vi "Main.vi"(8 "error in (no error)":errorcluster, 11 "ModuleAdmin":refnum<class "ModuleAdmin.lvclass">) -> ()   [LabVIEW 2018, in "SensorPlugins.lvlib"]
uses:
  SensorPlugins.lvlib
  <userlib>/NIST/ModuleAdminLib/ModuleAdmin/ModuleAdmin.lvclass
  C:/Program Files (x86)/National Instruments/LabVIEW 2018/user.lib/NIST/ModuleAdminLib/ModuleAdminBase/ModuleAdminBase.lvclass
  SensorBaseClass/SensorBase.lvclass
  C:/Program Files (x86)/National Instruments/LabVIEW 2018/user.lib/NIST/BaseClasses/BasePlugin_class/BasePlugin.lvclass
  SensorShared/clStopArgument.ctl
  <userlib>/NIST/ModuleAdminLib/ModuleAdmin/ModuleAdmin.lvclass/ModuleAdmin.ctl
  <userlib>/NIST/BaseClasses/BasePlugin_class/BasePlugin.lvclass/BasePlugin.ctl
  <vilib>/Utility/error.llb/DialogType.ctl
  <userlib>/NIST/ModuleAdminLib/ModuleAdmin/Accessors/Read ShowPanel_.vi
  <userlib>/NIST/ModuleAdminLib/ModuleAdmin/Accessors/Write ShowPanel_.vi
  <userlib>/NIST/BaseClasses/BasePlugin_class/Accessors/Write PluginIniFilePath.vi
  <userlib>/NIST/BaseClasses/BasePlugin_class/Accessors/Read PluginIniFilePath.vi
  <userlib>/NIST/ModuleAdminLib/ModuleAdmin/Accessors/Read CloneRegRef.vi
  <vilib>/Utility/error.llb/Error Cluster From Error Code.vi
  <vilib>/ErrorRing/Error Ring.xnode
  <userlib>/NIST/ModuleAdminLib/CloneRegistration/CloneRegistration.lvclass
  SensorShared/SensorShared.lvlib
  <userlib>/NIST/BaseClasses/Object_class/BaseObject.lvclass
  <userlib>/NIST/ModuleAdminLib/ModuleAdmin.lvlib
panel:
  out "error out":errorcluster
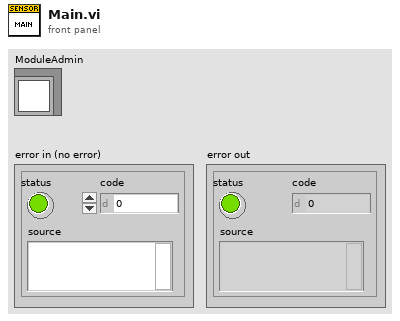
[diagram p1: front panel]
types:
  T1 = typedef "SensorShared.lvlib/clRequestEvents.ctl" = cluster{"StopRequest":refnum<user-event>, "PathToINI":refnum<user-event>, " LoadPlugin":refnum<user-event>, "ShowPanel":refnum<user-event>, "StartData":refnum<user-event>, "StopData":refnum<user-event>, "WriteConfig":refnum<user-event>, "ReadConfig":refnum<user-event>, "WriteEvtSignal":refnum<user-event>, "Configure":refnum<user-event>}
  T2 = typedef "SensorShared.lvlib/clBroadcastEvents.ctl" = cluster{"DidInit":refnum<user-event>, "StatusUpdate":refnum<user-event>, "ErrorReport":refnum<user-event>, "DidStop":refnum<user-event>, "PathToINI":refnum<user-event>, "SensorReport":refnum<user-event>, "SensorConfig":refnum<user-event>}
  T3 = typedef "SensorShared.lvlib/clStopArgument.ctl" = cluster{"Exit via Stop Module Req?":bool, "Wait for Module to stop?":bool, "ModuleAdmin":refnum<class "ModuleAdmin.lvclass">}
  T4 = enum32{"Invalid", "Standard", "Closed", "Hidden", "Minimized", "Maximized"}
  T5 = typedef "SensorShared.lvlib/clSensorData.ctl" = cluster{"SensorType":string, "SensorData":variant}
  T6 = typedef "DialogType.ctl" = u16
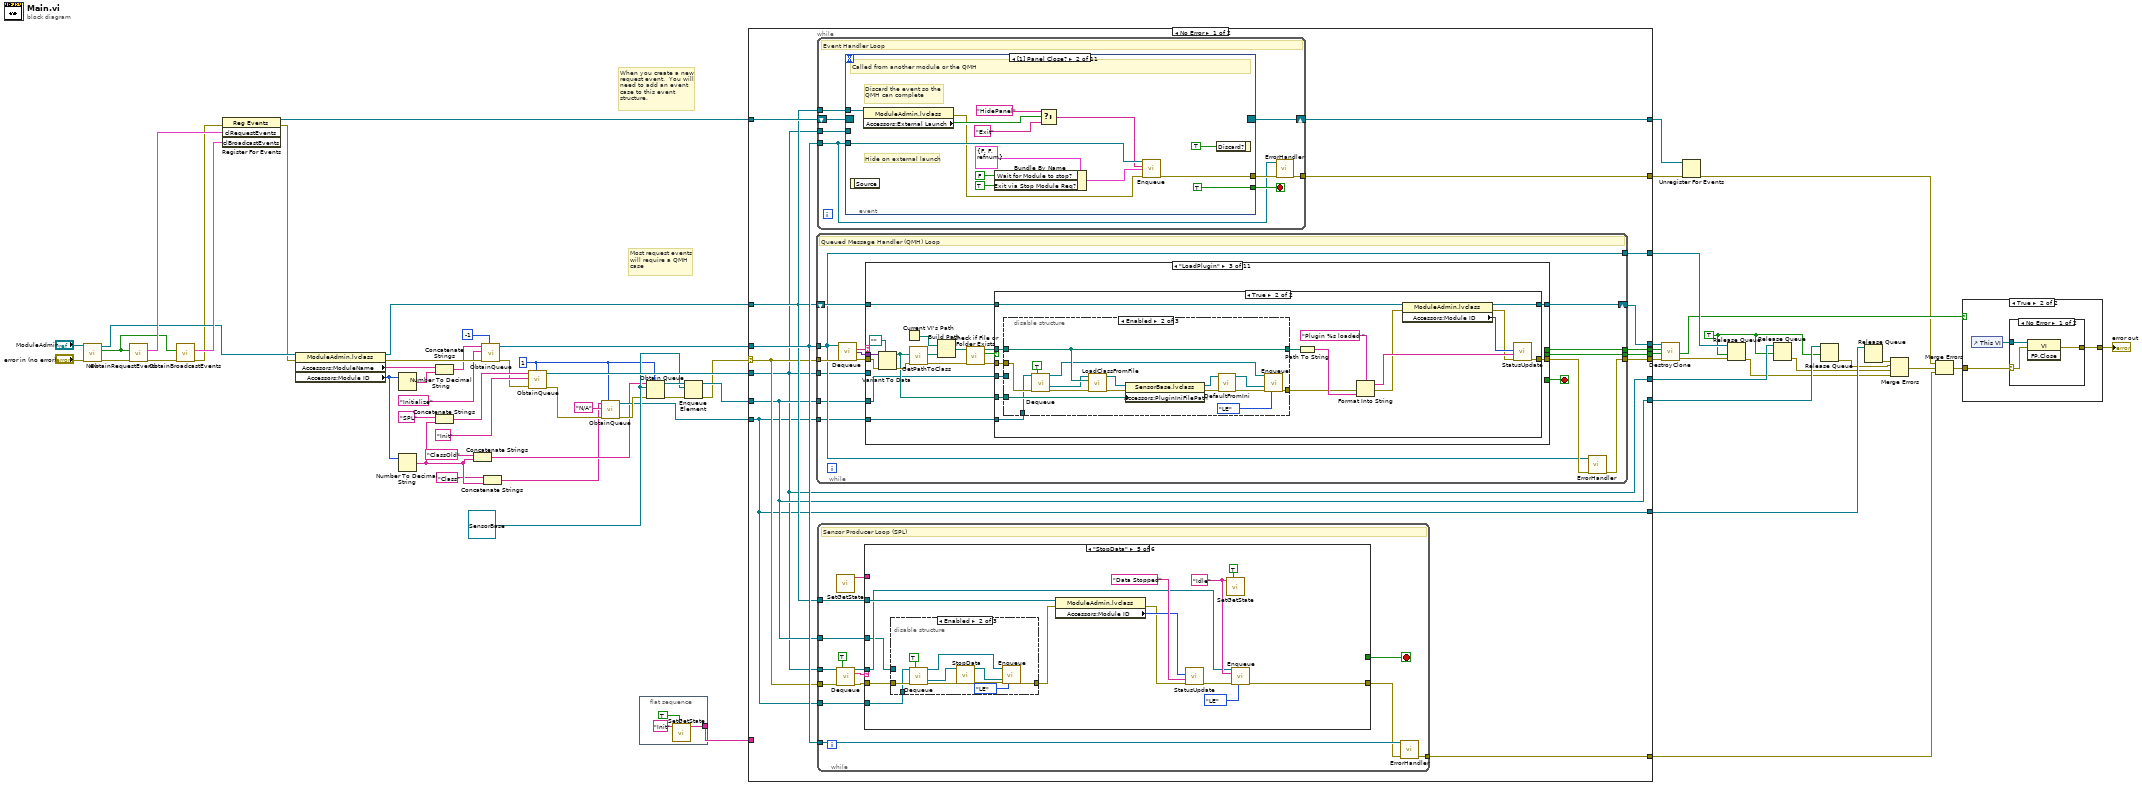
[diagram p0: block diagram]
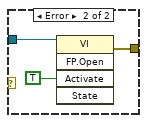
[diagram p3: hidden frame]
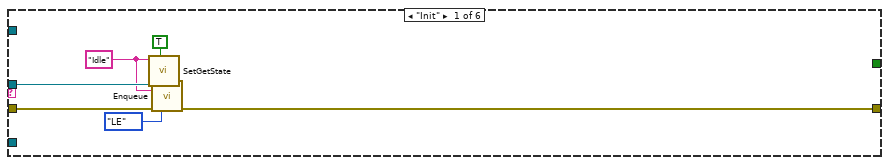
[diagram p4: hidden frame]
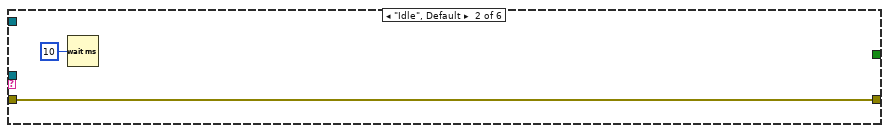
[diagram p5: hidden frame]
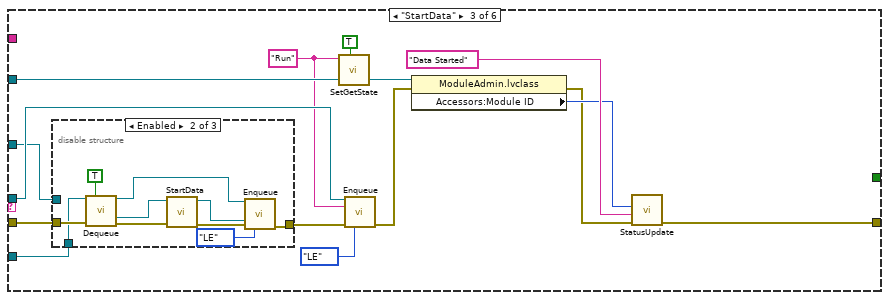
[diagram p6: hidden frame]
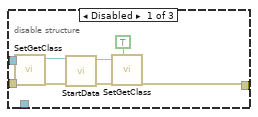
[diagram p7: hidden frame]
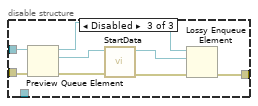
[diagram p8: hidden frame]
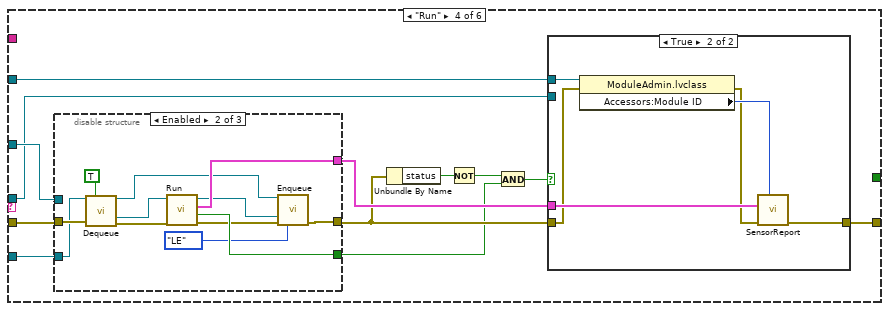
[diagram p9: hidden frame]
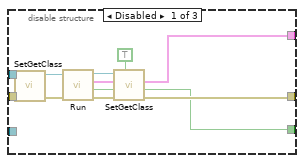
[diagram p10: hidden frame]
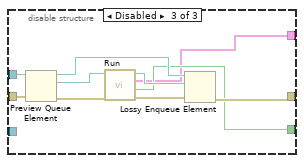
[diagram p11: hidden frame]
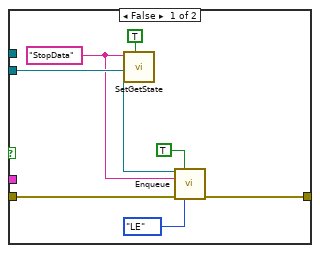
[diagram p12: hidden frame]
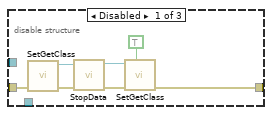
[diagram p13: hidden frame]
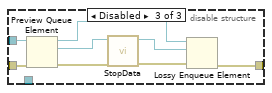
[diagram p14: hidden frame]
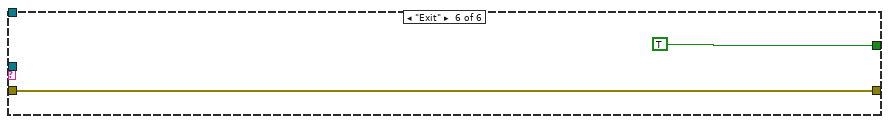
[diagram p15: hidden frame]
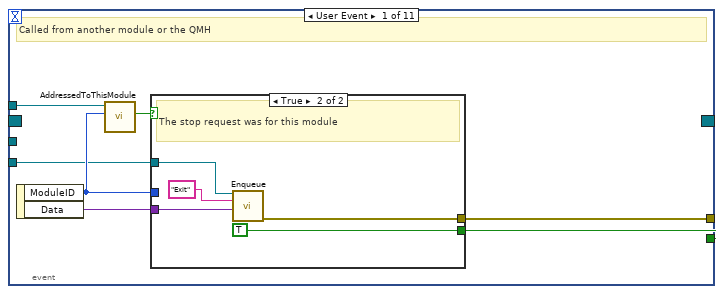
[diagram p16: hidden frame]
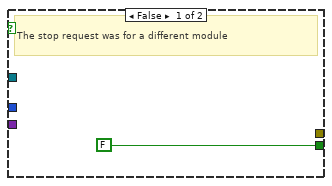
[diagram p17: hidden frame]
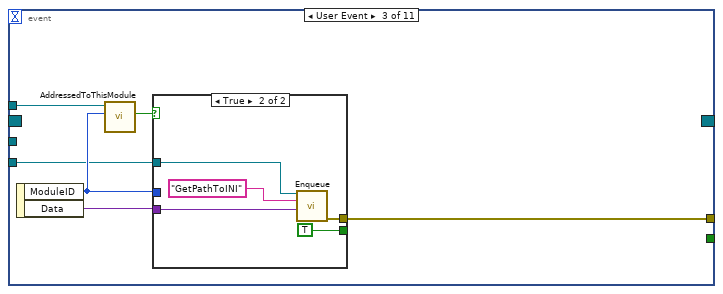
[diagram p18: hidden frame]
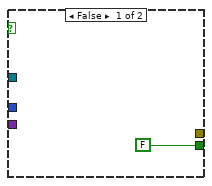
[diagram p19: hidden frame]
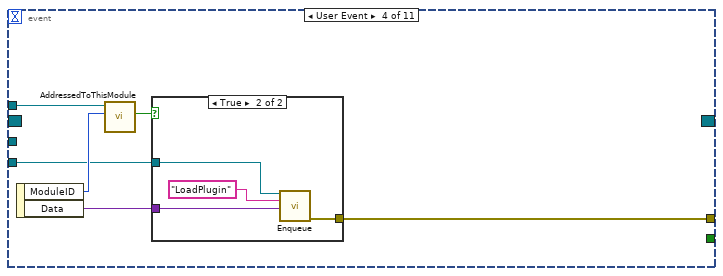
[diagram p20: hidden frame]
diagram:
  w16 = TRUE ("force destroy? (F)")
  w22 = refnum<class "SensorBase.lvclass"> refnum ("MyPlugins.lvlib:MyPluginsBase.lvclass")
  w14 = 1 ("Queue size (-1, unlimited)")
  # "Most request events\nwill require a QMH\ncase"
  # "When you create a new request event.  You will need to add an event case to this event structure."
  n1 = call <userlib>:"New.vi"("error in (no error)"="error in (no error)", "ModuleAdmin"="ModuleAdmin") -> ("error out"=w61:errorcluster, "First?"=w57:bool, "ModuleAdmin"=w42:refnum<class "ModuleAdmin.lvclass">)  [unwired: 6 in, 1 out]
  n2 = call "ObtainRequestEvents.vi"("error in (no error)"=w61, "CreateNew (F)"=w57) -> ("error out"=w56:errorcluster, "clRequestEvents"=w60:T1)  [unwired: 8 in]
  n3 = call "ObtainBroadcastEvents.vi"("error in (no error)"=w56, "CreateNew? (F)"=w57) -> ("error out"=w29:errorcluster, "clBroadcastEvents"=w55:T2)  [unwired: 8 in]
  n4 = register-events(error in=w29, w60, w55) -> (reference out=w54:refnum<event-registration>, error out=w28:errorcluster)  [unwired: 1 in]
  n5 = property class="ModuleAdmin.lvclass"(reference=w42, error in=w28) -> (reference out=w19:refnum<class "ModuleAdmin.lvclass">, error out=w44:errorcluster, "Accessors:ModuleName"=w40:string, "Accessors:Module ID"=w32:i32)
  n6 = Number To Decimal String(number=w32) -> (decimal integer string=w39:string)  [unwired: 1 in]
  n7 = Number To Decimal String(number=w32) -> (decimal integer string=w4:string)  [unwired: 1 in]
  n8 = Concatenate Strings(w40, w39) -> (w38:string)
  n9 = Concatenate Strings("SPL" ("Initial Message"), w4) -> (w34:string)
  n10 = Concatenate Strings("ClassOld" ("Initial Message"), w4) -> (w2:string)
  n11 = call "ObtainQueue.vi"("Queue size (-1, unlimited)"=-1, "error in (no error)"=w44, "Initial Message"="Initialize", "Queue Name"=w38) -> ("error out"=w33:errorcluster, "MessageQueue"=w59:refnum<queue>)  [unwired: 6 in]
  n12 = Concatenate Strings("Class" ("Initial Message"), w4) -> (w1:string)
  n13 = call "ObtainQueue.vi"("Queue size (-1, unlimited)"=w14, "error in (no error)"=w33, "Initial Message"="Init", "Queue Name"=w34) -> ("error out"=w15:errorcluster, "MessageQueue"=w30:refnum<queue>)  [unwired: 6 in]
  n14 = call "ObtainQueue.vi"("Queue size (-1, unlimited)"=w14, "error in (no error)"=w15, "Initial Message"="N/A", "Queue Name"=w1) -> ("error out"=w13:errorcluster, "MessageQueue"=w12:refnum<queue>)  [unwired: 6 in]
  n15 = flat-sequence {
    tunnel: [w64] -> w20
    frame #0 {
      n16 = call "SetGetState.vi"("Set (f)"=TRUE, "State In"="Init") -> ("State Out"=w64:string)  [unwired: 9 in]
    }
  }
  n17 = Obtain Queue(max queue size (-1, unlimited)=w14, name (unnamed)=w2, element data type=w22, error in (no error)=w13) -> (queue out=w24:refnum<queue>, error out=w26:errorcluster)  [unwired: 1 in, 1 out]
  n18 = Enqueue Element(queue=w24, element=w22, error in (no error)=w26) -> (queue out=w23:refnum<queue>, error out=w21:errorcluster)  [unwired: 1 in, 1 out]
  n19 = case shown="No Error" w21 {
    selector: w21 -> [w70 w737]
    tunnel: w59 -> [w74 w733]
    tunnel: w19 -> [w72 w734]
    tunnel: [w81 w735] -> w53
    tunnel: [w80 w733] -> w58
    tunnel: w54 -> [w79 w729]
    tunnel: [w78 w732] -> w51
    tunnel: [w77 _] -> w50
    tunnel: [w76 _] -> w49
    tunnel: [w75 _] -> w47
    tunnel: [w73 _] -> w27
    tunnel: [w71 w729] -> w46
    tunnel: w30 -> [w68 w726]
    tunnel: w23 -> [w69 w725]
    tunnel: w20 -> [_ _]
    tunnel: [w68 w726] -> w18
    tunnel: [w69 w725] -> w17
    tunnel: w12 -> [w67 w724]
    tunnel: [w67 w724] -> w10
    frame No Error {
      n20 = while {
        tunnel: w74 -> [w367]
        tunnel: w70 -> [w376]
        tunnel: [w369] -> w81
        tunnel: [w367] -> w80
        tunnel: [w371] -> w77
        tunnel: [w370] -> w76
        shift-right: [w366] -> w78
        shift-left: w72 -> [w372]
        tunnel: w69 -> [w365]
        tunnel: w68 -> [w364]
        tunnel: w67 -> [w363]
        stop <- w377 stop-if-true
        # "Queued Message Handler (QMH) Loop"
        n21 = call "Dequeue.vi"("MessageQueue"=w367, "error in (no error)"=w376) -> ("Message"=w374:string, "Message Data"=w373:variant, "error out"=w375:errorcluster)  [unwired: 9 in, 2 out]
        n22 = case shown="\"LoadPlugin\"" w374 {
          selector: w374 -> [_ _ _ _ _ _ _ _ _ _ w712]
          tunnel: [_ _ _ _ _ _ _ _ w680 _ _] -> w377
          tunnel: w372 -> [w403 w420 w428 w516 w540 w579 w617 w646 w681 w690 w715]
          tunnel: [w383 w414 w429 w517 w539 w577 w613 w644 w675 w691 w706] -> w368
          tunnel: w375 -> [w386 w423 w438 w514 w541 w573 w619 w640 w677 w688 w709]
          tunnel: w373 -> [_ w422 w440 _ _ w574 _ w641 w685 w698 _]
          tunnel: [_ _ _ _ _ _ _ _ w683 _ _] -> w371
          tunnel: [_ _ _ _ _ _ _ _ w682 _ _] -> w370
          tunnel: [w389 w419 w426 w513 w540 w578 w612 w645 w681 w686 w710] -> w366
          tunnel: w365 -> [_ _ w425 w510 w538 w570 w609 w637 _ _ _]
          tunnel: w364 -> [_ _ _ _ w537 w569 _ _ w679 _ _]
          tunnel: w363 -> [w381 _ w424 w509 w536 w568 w608 w636 _ _ _]
          frame "Initialize" {
            w382 = refnum<class "SensorBase.lvclass"> refnum ("MyPlugins.lvlib:MyPluginsBase.lvclass")
            # "Initialize is always called after ObtainQueue.vi is run"
            n23 = property class="ModuleAdmin.lvclass"(reference=w403, error in=w386) -> (reference out=w385:refnum<class "ModuleAdmin.lvclass">, error out=w400:errorcluster, "Accessors:Module ID"=w387:i32, "Accessors:ModuleName"=w391:string, "Accessors:ShowPanel_"=w379:bool, "Accessors:External Launch"=w380:bool)
            n24 = Compound Arithmetic op=OR(w379, invert w380) -> (w390:bool)
            n25 = Select(t=T4."Standard" ("Front Panel Window:State"), s=w390, f=T4."Hidden" ("Front Panel Window:State")) -> (s? t:f=w396:T4)
            n26 = invoke class="VI" method="FP.Open"(error in=w400, "State"=w396) -> (error out=w399:errorcluster)  [unwired: 3 in, 4 out]
            n27 = call <userlib>:"ModuleName.vi"("Name"=w391, "ModuleID"=w387) -> ("ModuleName"=w395:string)  [unwired: 9 in]
            n28 = property class="VI"(error in=w399, "Front Panel.Title"=w395) -> (reference out=w402:refnum<vi>, error out=w401:errorcluster)  [unwired: 1 in]
            n29 = invoke class="VI" method="FP.Center"(reference=w402, error in=w401) -> (error out=w392:errorcluster)  [unwired: 1 in, 2 out]
            n30 = case shown="True" w380 {
              tunnel: [w404 w410] -> w393
              tunnel: [w405 w407] -> w389
              tunnel: w392 -> [w404 w409]
              tunnel: w385 -> [w405 w406]
              frame False {
              }
              frame True {
                n31 = call <userlib>:"WaitOnModuleSync.vi"("error in (no error)"=w409, "ModuleAdmin"=w406) -> ("error out"=w411:errorcluster, "ModuleAdmin"=w408:refnum<class "ModuleAdmin.lvclass">)  [unwired: 8 in]
                n32 = call <userlib>:"WaitOnEventSync.vi"("error in (no error)"=w411, "ModuleAdmin"=w408) -> ("error out"=w410:errorcluster, "ModuleAdmin"=w407:refnum<class "ModuleAdmin.lvclass">)  [unwired: 8 in]
              }
            }
            n33 = call "DidInit.vi"("Init?"=TRUE, "error in (no error)"=w393, "ModuleAdmin"=w389) -> ("error out"=w384:errorcluster)  [unwired: 8 in]
            n34 = call "Enqueue.vi"("MessageQueue"=w381, "SensorBase in"=w382, "error in (no error)"=w384, "Type of Enqueue"=enum16{"Else", "LE"}."LE") -> ("error out"=w383:errorcluster)  [unwired: 10 in, 1 out]
            n35 = call "SetGetClass.vi"("Set (f)"=TRUE, "Class In"=w382) -> ()  [unwired: 9 in, 1 out]
          }
          frame "ShowPanel" {
            n36 = Variant To Data(error in=w423, type=TRUE, Variant=w422) -> (data=w416:bool, error out=w413:errorcluster)
            n37 = property class="ModuleAdmin.lvclass"(reference=w420, error in=w413, "Accessors:ShowPanel_"=w416) -> (reference out=w419:refnum<class "ModuleAdmin.lvclass">, error out=w412:errorcluster)
            n38 = Select(t=T4."Standard" ("Front Panel Window:State"), s=w416, f=T4."Hidden" ("Front Panel Window:State")) -> (s? t:f=w415:T4)
            n39 = property class="VI"(error in=w412, "FP.State"=w415) -> (error out=w414:errorcluster)  [unwired: 1 in, 1 out]
          }
          frame "LoadPlugin" {
            n40 = Variant To Data(error in=w438, type=path "", Variant=w440) -> (data=w427:path, error out=w437:errorcluster)
            n41 = Current VI's Path() -> (path=w435:path)
            n42 = call <userlib>:"GetPathToClass.vi"("error in (no error)"=w437, "configuration file path"=w427) -> ("error IO"=w433:errorcluster, "PathToClass"=w436:path)  [unwired: 8 in]
            n43 = Build Path(base path=w435, name or relative path=w436) -> (appended path=w434:path)
            n44 = call <vilib>:"Check if File or Folder Exists.vi"("error in (no error)"=w433, "path"=w434) -> ("error out"=w430:errorcluster, "file or folder exists?"=w432:bool, "dup path"=w431:path)  [unwired: 7 in]
            n45 = case shown="True" w432 {
              tunnel: w431 -> [w443 w455]
              tunnel: w430 -> [_ w467]
              tunnel: [w442 w458] -> w429
              tunnel: w428 -> [w441 w463]
              tunnel: w427 -> [_ w461]
              tunnel: [w441 w460] -> w426
              tunnel: w425 -> [_ w453]
              tunnel: w424 -> [_ w452]
              frame False {
                n46 = Path To String(path=w443) -> (string=w444:string)
                n47 = xnode "Error Ring"("parameter 0"=w444) -> ("error out"=w442:errorcluster)
              }
              frame True {
                n48 = disable-structure shown="Enabled" {
                  disable-tunnel: w467 -> [w478 w488 w502]
                  disable-tunnel: w461 -> [w474 w492 w506]
                  disable-tunnel: [w469 w483 w496] -> w457
                  disable-tunnel: w455 -> [w468 w489 w503]
                  disable-tunnel: [w468 w489 w503] -> w454
                  disable-tunnel: w453 -> [_ _ w499]
                  disable-tunnel: w452 -> [_ w487 _]
                  frame Disabled {
                    n49 = call-dynamic "LoadClassFromFile.vi"("error in (no error)"=w478, "class path"=w468, "reference in"=refnum<class "SensorBase.lvclass"> refnum ("MyPlugins.lvlib:MyPluginsBase.lvclass")) -> ("error out"=w475:errorcluster, "reference out"=w476:refnum<class "SensorBase.lvclass">)  [unwired: 7 in]
                    n50 = property class="SensorBase.lvclass"(reference=w476, error in=w475, "Accessors:PluginIniFilePath"=w474) -> (reference out=w472:refnum<class "SensorBase.lvclass">, error out=w470:errorcluster)
                    n51 = call-dynamic "DefaultFromIni.vi"("error in (no error)"=w470, "SensorBase in"=w472) -> ("error out"=w469:errorcluster, "SensorBase out"=w471:refnum<class "SensorBase.lvclass">)  [unwired: 8 in]
                    n52 = call "SetGetClass.vi"("Set (f)"=TRUE, "Class In"=w471) -> ()  [unwired: 9 in, 1 out]
                  }
                  frame Enabled {
                    n53 = call "Dequeue.vi"("MessageQueue"=w487, "Preview Queue (F)"=TRUE, "error in (no error)"=w488) -> ("MessageQueue"=w481:refnum<queue>, "SensorBase Out"=w486:refnum<class "SensorBase.lvclass">, "error out"=w479:errorcluster)  [unwired: 8 in, 2 out]
                    n54 = call-dynamic "LoadClassFromFile.vi"("error in (no error)"=w479, "class path"=w489, "reference in"=w486) -> ("error out"=w493:errorcluster, "reference out"=w494:refnum<class "SensorBase.lvclass">)  [unwired: 7 in]
                    n55 = property class="SensorBase.lvclass"(reference=w494, error in=w493, "Accessors:PluginIniFilePath"=w492) -> (reference out=w491:refnum<class "SensorBase.lvclass">, error out=w490:errorcluster)
                    n56 = call-dynamic "DefaultFromIni.vi"("error in (no error)"=w490, "SensorBase in"=w491) -> ("error out"=w485:errorcluster, "SensorBase out"=w484:refnum<class "SensorBase.lvclass">)  [unwired: 8 in]
                    n57 = call "Enqueue.vi"("MessageQueue"=w481, "SensorBase in"=w484, "error in (no error)"=w485, "Type of Enqueue"=enum16{"Else", "LE"}."LE") -> ("error out"=w483:errorcluster)  [unwired: 10 in, 1 out]
                  }
                  frame Disabled {
                    n58 = Preview Queue Element(queue=w499, error in (no error)=w502) -> (queue out=w495:refnum<queue>, element=w500:refnum<class "SensorBase.lvclass">, error out=w501:errorcluster)  [unwired: 1 in, 1 out]
                    n59 = call-dynamic "LoadClassFromFile.vi"("error in (no error)"=w501, "class path"=w503, "reference in"=w500) -> ("error out"=w507:errorcluster, "reference out"=w508:refnum<class "SensorBase.lvclass">)  [unwired: 7 in]
                    n60 = property class="SensorBase.lvclass"(reference=w508, error in=w507, "Accessors:PluginIniFilePath"=w506) -> (reference out=w505:refnum<class "SensorBase.lvclass">, error out=w504:errorcluster)
                    n61 = call-dynamic "DefaultFromIni.vi"("error in (no error)"=w504, "SensorBase in"=w505) -> ("error out"=w497:errorcluster, "SensorBase out"=w498:refnum<class "SensorBase.lvclass">)  [unwired: 8 in]
                    n62 = Lossy Enqueue Element(queue=w495, element=w498, error in (no error)=w497) -> (error out=w496:errorcluster)  [unwired: 3 out]
                  }
                }
                n63 = Path To String(path=w454) -> (string=w465:string)
                n64 = Format Into String(format string="Plugin %s loaded ", error in=w457, w465) -> (resulting string=w464:string, error out=w456:errorcluster)  [unwired: 1 in]
                n65 = property class="ModuleAdmin.lvclass"(reference=w463, error in=w456) -> (reference out=w460:refnum<class "ModuleAdmin.lvclass">, error out=w459:errorcluster, "Accessors:Module ID"=w462:i32)
                n66 = call "StatusUpdate.vi"("error in (no error)"=w459, "Status"=w464, "ModuleID"=w462) -> ("error out"=w458:errorcluster)  [unwired: 8 in]
              }
            }
          }
          frame "GetPathToINI" {
            n67 = disable-structure shown="Enabled" {
              disable-tunnel: [w522 w528 w534] -> w515
              disable-tunnel: w514 -> [w521 w527 w533]
              disable-tunnel: [w519 w529 w535] -> w512
              disable-tunnel: w510 -> [_ _ w531]
              disable-tunnel: w509 -> [_ w524 _]
              frame Disabled {
                n68 = call "SetGetClass.vi"() -> ("Class Out"=w520:refnum<class "SensorBase.lvclass">)  [unwired: 11 in]
                n69 = property class="SensorBase.lvclass"(reference=w520, error in=w521) -> (error out=w519:errorcluster, "Accessors:PluginIniFilePath"=w522:path)  [unwired: 1 out]
              }
              frame Enabled {
                n70 = call "Dequeue.vi"("MessageQueue"=w524, "Preview Queue (F)"=TRUE, "error in (no error)"=w527) -> ("SensorBase Out"=w525:refnum<class "SensorBase.lvclass">, "error out"=w526:errorcluster)  [unwired: 8 in, 3 out]
                n71 = property class="SensorBase.lvclass"(reference=w525, error in=w526) -> (error out=w529:errorcluster, "Accessors:PluginIniFilePath"=w528:path)  [unwired: 1 out]
              }
              frame Disabled {
                n72 = Preview Queue Element(queue=w531, error in (no error)=w533) -> (element=w530:refnum<class "SensorBase.lvclass">, error out=w532:errorcluster)  [unwired: 1 in, 2 out]
                n73 = property class="SensorBase.lvclass"(reference=w530, error in=w532) -> (error out=w535:errorcluster, "Accessors:PluginIniFilePath"=w534:path)  [unwired: 1 out]
              }
            }
            n74 = property class="ModuleAdmin.lvclass"(reference=w516, error in=w512) -> (reference out=w513:refnum<class "ModuleAdmin.lvclass">, error out=w511:errorcluster, "Accessors:Module ID"=w518:i32)
            n75 = call "PathToINIBroadcast.vi"("error in (no error)"=w511, "PathToINI"=w515, "ModuleID"=w518) -> ("error out"=w517:errorcluster)  [unwired: 8 in]
          }
          frame "Configure" {
            n76 = disable-structure shown="Enabled" {
              disable-tunnel: w541 -> [w545 w552 w567]
              disable-tunnel: [w542 w555 w561] -> w539
              disable-tunnel: w538 -> [_ _ w564]
              disable-tunnel: w537 -> [_ w553 w559]
              disable-tunnel: w536 -> [_ w549 _]
              frame Disabled {
                n77 = call "SetGetClass.vi"() -> ("Class Out"=w546:refnum<class "SensorBase.lvclass">)  [unwired: 11 in]
                n78 = call-dynamic "ConfigureDlg.vi"("error in (no error)"=w545, "PmuBase in"=w546) -> ("error out"=w542:errorcluster, "PmuBase out"=w544:refnum<class "SensorBase.lvclass">)  [unwired: 7 in, 1 out]
                n79 = call "SetGetClass.vi"("Set (f)"=TRUE, "Class In"=w544) -> ()  [unwired: 9 in, 1 out]
              }
              frame Enabled {
                n80 = call "Dequeue.vi"("MessageQueue"=w549, "Preview Queue (F)"=TRUE, "error in (no error)"=w552) -> ("MessageQueue"=w548:refnum<queue>, "SensorBase Out"=w550:refnum<class "SensorBase.lvclass">, "error out"=w551:errorcluster)  [unwired: 8 in, 2 out]
                n81 = call-dynamic "ConfigureDlg.vi"("error in (no error)"=w551, "PmuBase in"=w550) -> ("error out"=w557:errorcluster, "Changed"=w554:bool, "PmuBase out"=w556:refnum<class "SensorBase.lvclass">)  [unwired: 7 in]
                n82 = call "CheckOnIdle.vi"("DataMessageQueue"=w553, "ClassQueue"=w548, "error in (no error)"=w557, "ChangeOccured? (F)"=w554, "SensorBase in"=w556) -> ("Error Out"=w555:errorcluster)  [unwired: 4 in, 2 out]
              }
              frame Disabled {
                n83 = Preview Queue Element(queue=w564, error in (no error)=w567) -> (queue out=w558:refnum<queue>, element=w565:refnum<class "SensorBase.lvclass">, error out=w566:errorcluster)  [unwired: 1 in, 1 out]
                n84 = call-dynamic "ConfigureDlg.vi"("error in (no error)"=w566, "PmuBase in"=w565) -> ("error out"=w563:errorcluster, "Changed"=w560:bool, "PmuBase out"=w562:refnum<class "SensorBase.lvclass">)  [unwired: 7 in]
                n85 = call "CheckOnIdle.vi"("DataMessageQueue"=w559, "ClassQueue"=w558, "error in (no error)"=w563, "ChangeOccured? (F)"=w560, "SensorBase in"=w562) -> ("Error Out"=w561:errorcluster)  [unwired: 4 in, 2 out]
              }
            }
          }
          frame "WriteConfig" {
            n86 = disable-structure shown="Enabled" {
              disable-tunnel: w574 -> [w584 w597 w605]
              disable-tunnel: w573 -> [w583 w591 w607]
              disable-tunnel: [w580 w596 w602] -> w572
              disable-tunnel: w570 -> [_ _ w604]
              disable-tunnel: w569 -> [_ w593 w599]
              disable-tunnel: w568 -> [_ w588 _]
              frame Disabled {
                n87 = call "SetGetClass.vi"() -> ("Class Out"=w585:refnum<class "SensorBase.lvclass">)  [unwired: 11 in]
                n88 = call-dynamic "WriteConfig.vi"("error in (no error)"=w583, "Config"=w584, "SensorBase in"=w585) -> ("error out"=w580:errorcluster, "SensorBase out"=w582:refnum<class "SensorBase.lvclass">)  [unwired: 7 in]
                n89 = call "SetGetClass.vi"("Set (f)"=TRUE, "Class In"=w582) -> ()  [unwired: 9 in, 1 out]
              }
              frame Enabled {
                n90 = call "Dequeue.vi"("MessageQueue"=w588, "Preview Queue (F)"=TRUE, "error in (no error)"=w591) -> ("MessageQueue"=w586:refnum<queue>, "SensorBase Out"=w589:refnum<class "SensorBase.lvclass">, "error out"=w590:errorcluster)  [unwired: 8 in, 2 out]
                n91 = call-dynamic "WriteConfig.vi"("error in (no error)"=w590, "Config"=w597, "SensorBase in"=w589) -> ("error out"=w595:errorcluster, "SensorBase out"=w594:refnum<class "SensorBase.lvclass">)  [unwired: 7 in]
                n92 = call "CheckOnIdle.vi"("DataMessageQueue"=w593, "ClassQueue"=w586, "error in (no error)"=w595, "ChangeOccured? (F)"=TRUE, "SensorBase in"=w594) -> ("Error Out"=w596:errorcluster)  [unwired: 4 in, 2 out]
              }
              frame Disabled {
                n93 = Preview Queue Element(queue=w604, error in (no error)=w607) -> (element=w603:refnum<class "SensorBase.lvclass">, error out=w606:errorcluster)  [unwired: 1 in, 2 out]
                n94 = call-dynamic "WriteConfig.vi"("error in (no error)"=w606, "Config"=w605, "SensorBase in"=w603) -> ("error out"=w601:errorcluster, "SensorBase out"=w600:refnum<class "SensorBase.lvclass">)  [unwired: 7 in]
                n95 = call "CheckOnIdle.vi"("DataMessageQueue"=w599, "error in (no error)"=w601, "ChangeOccured? (F)"=TRUE, "SensorBase in"=w600) -> ("Error Out"=w602:errorcluster)  [unwired: 5 in, 2 out]
              }
            }
            n96 = property class="ModuleAdmin.lvclass"(reference=w579, error in=w572) -> (reference out=w578:refnum<class "ModuleAdmin.lvclass">, error out=w571:errorcluster, "Accessors:Module ID"=w576:i32)
            n97 = call "StatusUpdate.vi"("error in (no error)"=w571, "Status"="Configuration Received", "ModuleID"=w576) -> ("error out"=w577:errorcluster)  [unwired: 8 in]
          }
          frame "ReadConfig" {
            n98 = disable-structure shown="Enabled" {
              disable-tunnel: w619 -> [w622 w627 w632]
              disable-tunnel: [w621 w629 w635] -> w611
              disable-tunnel: [w620 w628 w634] -> w618
              disable-tunnel: w609 -> [_ w624 _]
              disable-tunnel: w608 -> [_ _ w631]
              frame Disabled {
                n99 = call "SetGetClass.vi"() -> ("Class Out"=w623:refnum<class "SensorBase.lvclass">)  [unwired: 11 in]
                n100 = call-dynamic "ReadConfig.vi"("error in (no error)"=w622, "SensorBase in"=w623) -> ("error out"=w621:errorcluster, "Config"=w620:variant)  [unwired: 7 in, 1 out]
              }
              frame Disabled {
                n101 = Preview Queue Element(queue=w624, error in (no error)=w627) -> (element=w625:refnum<class "SensorBase.lvclass">, error out=w626:errorcluster)  [unwired: 1 in, 2 out]
                n102 = call-dynamic "ReadConfig.vi"("error in (no error)"=w626, "SensorBase in"=w625) -> ("error out"=w629:errorcluster, "Config"=w628:variant)  [unwired: 7 in, 1 out]
              }
              frame Enabled {
                n103 = call "Dequeue.vi"("MessageQueue"=w631, "error in (no error)"=w632) -> ("SensorBase Out"=w630:refnum<class "SensorBase.lvclass">, "error out"=w633:errorcluster)  [unwired: 9 in, 3 out]
                n104 = call-dynamic "ReadConfig.vi"("error in (no error)"=w633, "SensorBase in"=w630) -> ("error out"=w635:errorcluster, "Config"=w634:variant)  [unwired: 7 in, 1 out]
              }
            }
            n105 = property class="ModuleAdmin.lvclass"(reference=w617, error in=w611) -> (reference out=w612:refnum<class "ModuleAdmin.lvclass">, error out=w610:errorcluster, "Accessors:Module ID"=w616:i32)
            n106 = call "SensorConfig.vi"("ModuleID"=w616, "error in (no error)"=w610, "Config"=w618) -> ("error out"=w615:errorcluster)  [unwired: 8 in]
            n107 = call "StatusUpdate.vi"("error in (no error)"=w615, "Status"="Config Transmitted", "ModuleID"=w616) -> ("error out"=w613:errorcluster)  [unwired: 8 in]
          }
          frame "WriteEvtSignal" {
            n108 = disable-structure shown="Enabled" {
              disable-tunnel: w641 -> [w651 w663 w672]
              disable-tunnel: w640 -> [w650 w662 w671]
              disable-tunnel: [w647 w655 w667] -> w639
              disable-tunnel: w637 -> [_ _ w670]
              disable-tunnel: w636 -> [_ w659 _]
              frame Disabled {
                n109 = call "SetGetClass.vi"() -> ("Class Out"=w652:refnum<class "SensorBase.lvclass">)  [unwired: 11 in]
                n110 = call-dynamic "WriteEvtSignal.vi"("error in (no error)"=w650, "EvtSignal"=w651, "SensorBase in"=w652) -> ("error out"=w647:errorcluster, "SensorBase out"=w649:refnum<class "SensorBase.lvclass">)  [unwired: 7 in]
                n111 = call "SetGetClass.vi"("Set (f)"=TRUE, "Class In"=w649) -> ()  [unwired: 9 in, 1 out]
              }
              frame Enabled {
                n112 = call "Dequeue.vi"("MessageQueue"=w659, "Preview Queue (F)"=TRUE, "error in (no error)"=w662) -> ("MessageQueue"=w654:refnum<queue>, "SensorBase Out"=w660:refnum<class "SensorBase.lvclass">, "error out"=w661:errorcluster)  [unwired: 8 in, 2 out]
                n113 = call-dynamic "WriteEvtSignal.vi"("error in (no error)"=w661, "EvtSignal"=w663, "SensorBase in"=w660) -> ("error out"=w656:errorcluster, "SensorBase out"=w653:refnum<class "SensorBase.lvclass">)  [unwired: 7 in]
                n114 = call "Enqueue.vi"("MessageQueue"=w654, "SensorBase in"=w653, "error in (no error)"=w656, "Type of Enqueue"=enum16{"Else", "LE"}."LE") -> ("error out"=w655:errorcluster)  [unwired: 10 in, 1 out]
              }
              frame Disabled {
                n115 = Preview Queue Element(queue=w670, error in (no error)=w671) -> (queue out=w664:refnum<queue>, element=w668:refnum<class "SensorBase.lvclass">, error out=w669:errorcluster)  [unwired: 1 in, 1 out]
                n116 = call-dynamic "WriteEvtSignal.vi"("error in (no error)"=w669, "EvtSignal"=w672, "SensorBase in"=w668) -> ("error out"=w666:errorcluster, "SensorBase out"=w665:refnum<class "SensorBase.lvclass">)  [unwired: 7 in]
                n117 = Enqueue Element(queue=w664, element=w665, error in (no error)=w666) -> (error out=w667:errorcluster)  [unwired: 1 in, 2 out]
              }
            }
            n118 = property class="ModuleAdmin.lvclass"(reference=w646, error in=w639) -> (reference out=w645:refnum<class "ModuleAdmin.lvclass">, error out=w638:errorcluster, "Accessors:Module ID"=w643:i32)
            n119 = call "StatusUpdate.vi"("error in (no error)"=w638, "Status"="Waveform Received", "ModuleID"=w643) -> ("error out"=w644:errorcluster)  [unwired: 8 in]
          }
          frame "Exit" {
            w674 = "Exit" ("State In")
            w680 = TRUE
            # "Called by the StopRequest event handler case"
            n120 = control-ref of="This VI"() -> (w684:refnum<vi>)
            n121 = call "HandleExit.vi"("error in (no error)"=w677, "VI Refnum"=w684, "StopArgument"=w685, "ModuleAdmin"=w681) -> ("error out"=w676:errorcluster, "Exit via Stop Module Req?"=w682:bool, "WaitForStop?"=w683:bool)  [unwired: 5 in]
            n122 = call "Enqueue.vi"("MessageQueue"=w679, "Priority (F)"=TRUE, "Message"=w674, "error in (no error)"=w676, "Type of Enqueue"=enum16{"Else", "LE"}."LE" ("Enum")) -> ("error out"=w675:errorcluster)  [unwired: 9 in, 1 out]
            n123 = call "SetGetState.vi"("Set (f)"=w680, "State In"=w674) -> ()  [unwired: 9 in, 1 out]
          }
          frame "Error" {
            n124 = property class="ModuleAdmin.lvclass"(reference=w690, error in=w688) -> (reference out=w689:refnum<class "ModuleAdmin.lvclass">, error out=w687:errorcluster, "Accessors:External Launch"=w694:bool, "Accessors:Module ID"=w692:i32)
            n125 = Variant To Data(error in=w687, type=errorcluster {"status"=FALSE, "code"=0, "source"=""} ("error constant"), Variant=w698) -> (data=w693:errorcluster, error out=w696:errorcluster)
            n126 = call "ReportError.vi"("error in (no error)"=w696, "ErrorReported"=w693, "ModuleID"=w692) -> ("error out"=w695:errorcluster)  [unwired: 8 in]
            n127 = case shown="False" w694 {
              tunnel: w695 -> [w703 w705]
              tunnel: w693 -> [w702 _]
              tunnel: [w701 w705] -> w691
              tunnel: w689 -> [w700 w704]
              tunnel: [w699 w704] -> w686
              frame False {
                # "Todo:  Add an event to ask the user\nIf the module should stop or continue"
                # "Stand alone: now, force an exit"
                n128 = call "StopRequest.vi"("error in (no error)"=w703, "ModuleAdminIn"=w700) -> ("error out"=w701:errorcluster, "ModuleAdminOut"=w699:refnum<class "ModuleAdmin.lvclass">)  [unwired: 7 in, 1 out]
                n129 = call <vilib>:"Simple Error Handler.vi"("error in (no error)"=w702) -> ()  [unwired: 4 in, 5 out]
              }
              frame True {
                # "Externally launched modules only broadcast the error msg"
              }
            }
          }
          frame Default {
            # "Called only if a message was queued and no QMH case was created"
            n130 = property class="ModuleAdmin.lvclass"(reference=w715, error in=w709) -> (reference out=w710:refnum<class "ModuleAdmin.lvclass">, error out=w707:errorcluster, "Accessors:Module ID"=w714:i32, "Accessors:ModuleName"=w711:string)
            n131 = call <userlib>:"ModuleName.vi"("Name"=w711, "ModuleID"=w714) -> ("ModuleName"=w713:string)  [unwired: 9 in]
            n132 = xnode "Error Ring"("parameter 0"=w712, "parameter 1"=w713) -> ("error out"=w708:errorcluster)
            n133 = Merge Errors(w707, w708) -> (w706:errorcluster)
          }
        }
        n134 = call "ErrorHandler.vi"("error in (no error)"=w368, "MessageQueue"=w367) -> ("error out"=w369:errorcluster)  [unwired: 8 in, 1 out]
      }
      n135 = while {
        tunnel: w74 -> [w235]
        shift-right: [w239] -> w71
        shift-left: w79 -> [w240]
        tunnel: w72 -> [w238]
        tunnel: [w236] -> w75
        tunnel: w68 -> [w234]
        stop <- w241 stop-if-true
        # "Event Handler Loop"
        n136 = event shown="[1] Panel Close?" {
          selector: w240 -> [_ _ _ _ _ _ _ _ _ _ _]
          dyn-events: [_ _ _ _ _ _ _ _ _ _ _] -> w239
          timeout: _ -> [_ _ _ _ _ _ _ _ _ _ _]
          tunnel: w235 -> [w245 w268 w271 w282 w292 w302 w312 w322 w332 _ _]
          tunnel: [w244 TRUE _ _ _ _ _ _ _ _ _] -> w241
          tunnel: w238 -> [w248 w262 w270 w286 w296 w306 w316 w326 w336 w346 w357]
          tunnel: [w243 w266 w269 w283 w293 w303 w313 w323 w333 w342 w353] -> w237
          tunnel: w234 -> [_ _ _ _ _ _ _ _ _ w341 w352]
          event User Event {
            # "Called from another module or the QMH"
            n137 = event-data() -> ("ModuleID"=w246:i32, "Data"=w242:variant)  [unwired: 1 in]
            n138 = call <userlib>:"AddressedToThisModule.vi"("ModuleID"=w246, "ModuleAdmin"=w248) -> ("AddressedToThisInstance?"=w247:bool)  [unwired: 8 in, 1 out]
            n139 = case shown="True" w247 {
              tunnel: w246 -> [_ _]
              tunnel: w245 -> [_ w254]
              tunnel: [FALSE TRUE] -> w244
              tunnel: [_ w252] -> w243
              tunnel: w242 -> [_ w250]
              frame False {
                # "The stop request was for a different module"
              }
              frame True {
                # "The stop request was for this module"
                n140 = call "Enqueue.vi"("MessageQueue"=w254, "Message"="Exit", "Message Data"=w250) -> ("error out"=w252:errorcluster)  [unwired: 11 in, 1 out]
              }
            }
          }
          event Panel Close? {
            # "Hide on external launch"
            # "Discard the event so the QMH can complete"
            # "Called from another module or the QMH"
            n141 = event-data() -> ()  [unwired: 1 in, 1 out]
            n142 = property class="ModuleAdmin.lvclass"(reference=w262) -> (error out=w255:errorcluster, "Accessors:External Launch"=w257:bool)  [unwired: 1 in, 1 out]
            n143 = Bundle By Name(cluster=T3 {"Exit via Stop Module Req?"=FALSE, "Wait for Module to stop?"=FALSE, "ModuleAdmin"=refnum} ("Stop Argument"), "Wait for Module to stop?"=FALSE, "Exit via Stop Module Req?"=TRUE) -> (w263:T3)
            n144 = Select(t="HidePanel", s=w257, f="Exit" ("Message")) -> (s? t:f=w259:string)
            n145 = call "Enqueue.vi"("MessageQueue"=w268, "Message"=w259, "Message Data"=w263, "error in (no error)"=w255) -> ("error out"=w266:errorcluster)  [unwired: 10 in, 1 out]
            n146 = event-data("Discard?"=TRUE) -> ()  [unwired: 1 in, 1 out]
          }
          event User Event {
            n147 = event-data() -> ("ModuleID"=w272:i32, "Data"=w273:variant)  [unwired: 1 in]
            n148 = call <userlib>:"AddressedToThisModule.vi"("ModuleID"=w272, "ModuleAdmin"=w270) -> ("AddressedToThisInstance?"=w274:bool)  [unwired: 8 in, 1 out]
            n149 = case shown="True" w274 {
              tunnel: w272 -> [_ _]
              tunnel: w271 -> [_ w280]
              tunnel: [FALSE TRUE] -> _
              tunnel: [_ w278] -> w269
              tunnel: w273 -> [_ w276]
              frame False {
                # "The stop request was for a different module"
              }
              frame True {
                # "The stop request was for this module"
                n150 = call "Enqueue.vi"("MessageQueue"=w280, "Message"="GetPathToINI", "Message Data"=w276) -> ("error out"=w278:errorcluster)  [unwired: 11 in, 1 out]
              }
            }
          }
          event User Event {
            n151 = event-data() -> ("ModuleID"=w285:i32, "Data"=w281:variant)  [unwired: 1 in]
            n152 = call <userlib>:"AddressedToThisModule.vi"("ModuleID"=w285, "ModuleAdmin"=w286) -> ("AddressedToThisInstance?"=w284:bool)  [unwired: 8 in, 1 out]
            n153 = case shown="True" w284 {
              tunnel: [_ w287] -> w283
              tunnel: w282 -> [_ w290]
              tunnel: w281 -> [_ w288]
              frame False {
              }
              frame True {
                n154 = call "Enqueue.vi"("MessageQueue"=w290, "Message"="LoadPlugin", "Message Data"=w288) -> ("error out"=w287:errorcluster)  [unwired: 11 in, 1 out]
              }
            }
          }
          event User Event {
            n155 = event-data() -> ("ModuleID"=w295:i32, "Data"=w291:variant)  [unwired: 1 in]
            n156 = call <userlib>:"AddressedToThisModule.vi"("ModuleID"=w295, "ModuleAdmin"=w296) -> ("AddressedToThisInstance?"=w294:bool)  [unwired: 8 in, 1 out]
            n157 = case shown="True" w294 {
              tunnel: [_ w297] -> w293
              tunnel: w292 -> [_ w300]
              tunnel: w291 -> [_ w298]
              frame False {
              }
              frame True {
                n158 = call "Enqueue.vi"("MessageQueue"=w300, "Message"="ShowPanel", "Message Data"=w298) -> ("error out"=w297:errorcluster)  [unwired: 11 in, 1 out]
              }
            }
          }
          event User Event {
            n159 = event-data() -> ("ModuleID"=w305:i32, "Data"=w301:variant)  [unwired: 1 in]
            n160 = call <userlib>:"AddressedToThisModule.vi"("ModuleID"=w305, "ModuleAdmin"=w306) -> ("AddressedToThisInstance?"=w304:bool)  [unwired: 8 in, 1 out]
            n161 = case shown="True" w304 {
              tunnel: [_ w307] -> w303
              tunnel: w302 -> [_ w310]
              tunnel: w301 -> [_ w308]
              frame False {
              }
              frame True {
                n162 = call "Enqueue.vi"("MessageQueue"=w310, "Message"="Configure", "Message Data"=w308) -> ("error out"=w307:errorcluster)  [unwired: 11 in, 1 out]
              }
            }
          }
          event User Event {
            n163 = event-data() -> ("ModuleID"=w315:i32, "Data"=w311:variant)  [unwired: 1 in]
            n164 = call <userlib>:"AddressedToThisModule.vi"("ModuleID"=w315, "ModuleAdmin"=w316) -> ("AddressedToThisInstance?"=w314:bool)  [unwired: 8 in, 1 out]
            n165 = case shown="True" w314 {
              tunnel: [_ w317] -> w313
              tunnel: w312 -> [_ w320]
              tunnel: w311 -> [_ w318]
              frame False {
              }
              frame True {
                n166 = call "Enqueue.vi"("MessageQueue"=w320, "Message"="WriteConfig", "Message Data"=w318) -> ("error out"=w317:errorcluster)  [unwired: 11 in, 1 out]
              }
            }
          }
          event User Event {
            n167 = event-data() -> ("ModuleID"=w325:i32, "Data"=w321:variant)  [unwired: 1 in]
            n168 = call <userlib>:"AddressedToThisModule.vi"("ModuleID"=w325, "ModuleAdmin"=w326) -> ("AddressedToThisInstance?"=w324:bool)  [unwired: 8 in, 1 out]
            n169 = case shown="True" w324 {
              tunnel: [_ w327] -> w323
              tunnel: w322 -> [_ w330]
              tunnel: w321 -> [_ w328]
              frame False {
              }
              frame True {
                n170 = call "Enqueue.vi"("MessageQueue"=w330, "Message"="ReadConfig", "Message Data"=w328) -> ("error out"=w327:errorcluster)  [unwired: 11 in, 1 out]
              }
            }
          }
          event User Event {
            n171 = event-data() -> ("ModuleID"=w335:i32, "Data"=w331:variant)  [unwired: 1 in]
            n172 = call <userlib>:"AddressedToThisModule.vi"("ModuleID"=w335, "ModuleAdmin"=w336) -> ("AddressedToThisInstance?"=w334:bool)  [unwired: 8 in, 1 out]
            n173 = case shown="True" w334 {
              tunnel: [_ w337] -> w333
              tunnel: w332 -> [_ w340]
              tunnel: w331 -> [_ w338]
              frame False {
              }
              frame True {
                n174 = call "Enqueue.vi"("MessageQueue"=w340, "Message"="WriteEvtSignal", "Message Data"=w338) -> ("error out"=w337:errorcluster)  [unwired: 11 in, 1 out]
              }
            }
          }
          event User Event {
            n175 = event-data() -> ("ModuleID"=w345:i32, "Data"=w343:variant)  [unwired: 1 in]
            n176 = call <userlib>:"AddressedToThisModule.vi"("ModuleID"=w345, "ModuleAdmin"=w346) -> ("AddressedToThisInstance?"=w344:bool)  [unwired: 8 in, 1 out]
            n177 = case shown="True" w344 {
              tunnel: w341 -> [_ w350]
              tunnel: w343 -> [_ _]
              tunnel: [_ w348] -> w342
              frame False {
              }
              frame True {
                w349 = "StartData" ("State In")
                n178 = call "SetGetState.vi"("Set (f)"=TRUE, "State In"=w349) -> ()  [unwired: 9 in, 1 out]
                n179 = call "Enqueue.vi"("MessageQueue"=w350, "Message"=w349, "Type of Enqueue"=enum16{"Else", "LE"}."LE" ("Enum")) -> ("error out"=w348:errorcluster)  [unwired: 11 in, 1 out]
              }
            }
          }
          event User Event {
            n180 = event-data() -> ("ModuleID"=w356:i32, "Data"=w354:variant)  [unwired: 1 in]
            n181 = call <userlib>:"AddressedToThisModule.vi"("ModuleID"=w356, "ModuleAdmin"=w357) -> ("AddressedToThisInstance?"=w355:bool)  [unwired: 8 in, 1 out]
            n182 = case shown="True" w355 {
              tunnel: w352 -> [_ w361]
              tunnel: w354 -> [_ _]
              tunnel: [_ w360] -> w353
              frame False {
              }
              frame True {
                w359 = "StopData" ("State In")
                n183 = call "SetGetState.vi"("Set (f)"=TRUE, "State In"=w359) -> ()  [unwired: 9 in, 1 out]
                n184 = call "Enqueue.vi"("MessageQueue"=w361, "Message"=w359, "Type of Enqueue"=enum16{"Else", "LE"}."LE" ("Enum")) -> ("error out"=w360:errorcluster)  [unwired: 11 in, 1 out]
              }
            }
          }
        }
        n185 = call "ErrorHandler.vi"("error in (no error)"=w237, "MessageQueue"=w235) -> ("error out"=w236:errorcluster)  [unwired: 8 in, 1 out]
      }
      n186 = while {
        tunnel: w70 -> [w89]
        tunnel: w74 -> [w93]
        tunnel: [w92] -> w73
        tunnel: w72 -> [w90]
        tunnel: w68 -> [w87]
        tunnel: w69 -> [w84]
        tunnel: w67 -> [w82]
        stop <- w94 stop-if-true
        # "Sensor Producer Loop (SPL)"
        n187 = call "SetGetState.vi"() -> ("State Out"=w95:string)  [unwired: 11 in]
        n188 = call "Dequeue.vi"("MessageQueue"=w87, "Preview Queue (F)"=TRUE ("Preview Queue"), "error in (no error)"=w89) -> ("MessageQueue"=w86:refnum<queue>, "Message"=w83:string, "error out"=w88:errorcluster)  [unwired: 8 in, 2 out]
        n189 = case shown="\"StopData\"" w83 {
          tunnel: [_ _ _ _ _ TRUE] -> w94
          tunnel: [w99 w103 w115 w150 w202 w232] -> w91
          tunnel: w88 -> [w100 w103 w109 w152 w207 w232]
          tunnel: w90 -> [_ _ w114 w151 w205 _]
          tunnel: w86 -> [w98 _ w112 w142 w200 _]
          tunnel: w84 -> [_ _ w110 w143 w197 _]
          tunnel: w95 -> [_ _ _ _ _ _]
          tunnel: w82 -> [_ _ w104 w141 w195 _]
          frame "Init" {
            w97 = "Idle" ("State In")
            n190 = call "SetGetState.vi"("Set (f)"=TRUE, "State In"=w97) -> ()  [unwired: 9 in, 1 out]
            n191 = call "Enqueue.vi"("MessageQueue"=w98, "Message"=w97, "error in (no error)"=w100, "Type of Enqueue"=enum16{"Else", "LE"}."LE" ("Enum")) -> ("error out"=w99:errorcluster)  [unwired: 10 in, 1 out]
          }
          frame "Idle", Default {
            n192 = Wait (ms)(milliseconds to wait=u32 10) -> ()  [unwired: 1 out]
          }
          frame "StartData" {
            w111 = "Run" ("State In")
            n193 = disable-structure shown="Enabled" {
              disable-tunnel: w109 -> [w119 w132 w137]
              disable-tunnel: [w118 w129 w135] -> w108
              disable-tunnel: w110 -> [_ _ w139]
              disable-tunnel: w104 -> [_ w126 _]
              frame Disabled {
                n194 = call "SetGetClass.vi"() -> ("Class Out"=w122:refnum<class "SensorBase.lvclass">)  [unwired: 11 in]
                n195 = call-dynamic "StartData.vi"("error in (no error)"=w119, "Class In"=w122) -> ("error out"=w118:errorcluster, "Class Out"=w121:refnum<class "SensorBase.lvclass">)  [unwired: 8 in]
                n196 = call "SetGetClass.vi"("Set (f)"=TRUE, "Class In"=w121) -> ()  [unwired: 9 in, 1 out]
              }
              frame Enabled {
                n197 = call "Dequeue.vi"("MessageQueue"=w126, "Preview Queue (F)"=TRUE, "error in (no error)"=w132) -> ("MessageQueue"=w123:refnum<queue>, "SensorBase Out"=w130:refnum<class "SensorBase.lvclass">, "error out"=w131:errorcluster)  [unwired: 8 in, 2 out]
                n198 = call-dynamic "StartData.vi"("error in (no error)"=w131, "Class In"=w130) -> ("error out"=w128:errorcluster, "Class Out"=w127:refnum<class "SensorBase.lvclass">)  [unwired: 8 in]
                n199 = call "Enqueue.vi"("MessageQueue"=w123, "SensorBase in"=w127, "error in (no error)"=w128, "Type of Enqueue"=enum16{"Else", "LE"}."LE") -> ("error out"=w129:errorcluster)  [unwired: 10 in, 1 out]
              }
              frame Disabled {
                n200 = Preview Queue Element(queue=w139, error in (no error)=w137) -> (queue out=w134:refnum<queue>, element=w138:refnum<class "SensorBase.lvclass">, error out=w140:errorcluster)  [unwired: 1 in, 1 out]
                n201 = call-dynamic "StartData.vi"("error in (no error)"=w140, "Class In"=w138) -> ("error out"=w136:errorcluster, "Class Out"=w133:refnum<class "SensorBase.lvclass">)  [unwired: 8 in]
                n202 = Lossy Enqueue Element(queue=w134, element=w133, error in (no error)=w136) -> (error out=w135:errorcluster)  [unwired: 3 out]
              }
            }
            n203 = call "SetGetState.vi"("Set (f)"=TRUE, "State In"=w111) -> ()  [unwired: 9 in, 1 out]
            n204 = call "Enqueue.vi"("MessageQueue"=w112, "Message"=w111, "error in (no error)"=w108, "Type of Enqueue"=enum16{"Else", "LE"}."LE" ("Enum")) -> ("error out"=w107:errorcluster)  [unwired: 10 in, 1 out]
            n205 = property class="ModuleAdmin.lvclass"(reference=w114, error in=w107) -> (error out=w106:errorcluster, "Accessors:Module ID"=w113:i32)  [unwired: 1 out]
            n206 = call "StatusUpdate.vi"("error in (no error)"=w106, "Status"="Data Started", "ModuleID"=w113) -> ("error out"=w115:errorcluster)  [unwired: 8 in]
          }
          frame "Run" {
            n207 = disable-structure shown="Enabled" {
              disable-tunnel: w152 -> [w156 w168 w175]
              disable-tunnel: [w155 w170 w172] -> w149
              disable-tunnel: [w154 w163 w176] -> w148
              disable-tunnel: [w153 w171 w173] -> w146
              disable-tunnel: w143 -> [_ _ w174]
              disable-tunnel: w141 -> [_ w167 _]
              frame Disabled {
                n208 = call "SetGetClass.vi"() -> ("Class Out"=w159:refnum<class "SensorBase.lvclass">)  [unwired: 11 in]
                n209 = call-dynamic "Run.vi"("error in (no error)"=w156, "SensorBase in"=w159) -> ("error out"=w154:errorcluster, "DataValid"=w153:bool, "clSensorData"=w155:T5, "SensorBase out"=w158:refnum<class "SensorBase.lvclass">)  [unwired: 6 in]
                n210 = call "SetGetClass.vi"("Set (f)"=TRUE, "Class In"=w158) -> ()  [unwired: 9 in, 1 out]
              }
              frame Enabled {
                n211 = call "Dequeue.vi"("MessageQueue"=w167, "Preview Queue (F)"=TRUE, "error in (no error)"=w168) -> ("MessageQueue"=w160:refnum<queue>, "SensorBase Out"=w165:refnum<class "SensorBase.lvclass">, "error out"=w169:errorcluster)  [unwired: 8 in, 2 out]
                n212 = call-dynamic "Run.vi"("error in (no error)"=w169, "SensorBase in"=w165) -> ("error out"=w164:errorcluster, "DataValid"=w171:bool, "clSensorData"=w170:T5, "SensorBase out"=w161:refnum<class "SensorBase.lvclass">)  [unwired: 6 in]
                n213 = call "Enqueue.vi"("MessageQueue"=w160, "SensorBase in"=w161, "error in (no error)"=w164, "Type of Enqueue"=enum16{"Else", "LE"}."LE") -> ("error out"=w163:errorcluster)  [unwired: 10 in, 1 out]
              }
              frame Disabled {
                n214 = Preview Queue Element(queue=w174, error in (no error)=w175) -> (queue out=w181:refnum<queue>, element=w177:refnum<class "SensorBase.lvclass">, error out=w180:errorcluster)  [unwired: 1 in, 1 out]
                n215 = call-dynamic "Run.vi"("error in (no error)"=w180, "SensorBase in"=w177) -> ("error out"=w179:errorcluster, "DataValid"=w173:bool, "clSensorData"=w172:T5, "SensorBase out"=w178:refnum<class "SensorBase.lvclass">)  [unwired: 6 in]
                n216 = Lossy Enqueue Element(queue=w181, element=w178, error in (no error)=w179) -> (error out=w176:errorcluster)  [unwired: 3 out]
              }
            }
            n217 = Unbundle By Name(w148) -> ("status"=w147:bool)
            n218 = Not(x=w147) -> (.not. x?=w144:bool)
            n219 = And(x=w144, y=w146) -> (x .and. y?=w145:bool)
            n220 = case shown="True" w145 {
              tunnel: w151 -> [_ w194]
              tunnel: [w186 w193] -> w150
              tunnel: w149 -> [_ w191]
              tunnel: w148 -> [w187 w190]
              tunnel: w142 -> [w185 _]
              frame False {
                w183 = "StopData" ("State In")
                n221 = call "SetGetState.vi"("Set (f)"=TRUE, "State In"=w183) -> ()  [unwired: 9 in, 1 out]
                n222 = call "Enqueue.vi"("MessageQueue"=w185, "Priority (F)"=TRUE, "Message"=w183, "error in (no error)"=w187, "Type of Enqueue"=enum16{"Else", "LE"}."LE" ("Enum")) -> ("error out"=w186:errorcluster)  [unwired: 9 in, 1 out]
              }
              frame True {
                n223 = property class="ModuleAdmin.lvclass"(reference=w194, error in=w190) -> (error out=w189:errorcluster, "Accessors:Module ID"=w192:i32)  [unwired: 1 out]
                n224 = call "SensorReport.vi"("ModuleID"=w192, "error in (no error)"=w189, "clSensorData"=w191) -> ("error out"=w193:errorcluster)  [unwired: 8 in]
              }
            }
          }
          frame "StopData" {
            w201 = "Idle" ("State In")
            n225 = disable-structure shown="Enabled" {
              disable-tunnel: w207 -> [w213 w223 w227]
              disable-tunnel: [w209 w219 w226] -> w199
              disable-tunnel: w197 -> [_ _ w224]
              disable-tunnel: w195 -> [_ w222 _]
              frame Disabled {
                n226 = call "SetGetClass.vi"() -> ("Class Out"=w212:refnum<class "SensorBase.lvclass">)  [unwired: 11 in]
                n227 = call-dynamic "StopData.vi"("error in (no error)"=w213, "Class In"=w212) -> ("error out"=w209:errorcluster, "Class Out"=w211:refnum<class "SensorBase.lvclass">)  [unwired: 8 in]
                n228 = call "SetGetClass.vi"("Set (f)"=TRUE, "Class In"=w211) -> ()  [unwired: 9 in, 1 out]
              }
              frame Enabled {
                n229 = call "Dequeue.vi"("MessageQueue"=w222, "Preview Queue (F)"=TRUE, "error in (no error)"=w223) -> ("MessageQueue"=w216:refnum<queue>, "SensorBase Out"=w217:refnum<class "SensorBase.lvclass">, "error out"=w221:errorcluster)  [unwired: 8 in, 2 out]
                n230 = call-dynamic "StopData.vi"("error in (no error)"=w221, "Class In"=w217) -> ("error out"=w220:errorcluster, "Class Out"=w218:refnum<class "SensorBase.lvclass">)  [unwired: 8 in]
                n231 = call "Enqueue.vi"("MessageQueue"=w216, "SensorBase in"=w218, "error in (no error)"=w220, "Type of Enqueue"=enum16{"Else", "LE"}."LE") -> ("error out"=w219:errorcluster)  [unwired: 10 in, 1 out]
              }
              frame Disabled {
                n232 = Preview Queue Element(queue=w224, error in (no error)=w227) -> (queue out=w228:refnum<queue>, element=w231:refnum<class "SensorBase.lvclass">, error out=w230:errorcluster)  [unwired: 1 in, 1 out]
                n233 = call-dynamic "StopData.vi"("error in (no error)"=w230, "Class In"=w231) -> ("error out"=w229:errorcluster, "Class Out"=w225:refnum<class "SensorBase.lvclass">)  [unwired: 8 in]
                n234 = Lossy Enqueue Element(queue=w228, element=w225, error in (no error)=w229) -> (error out=w226:errorcluster)  [unwired: 3 out]
              }
            }
            n235 = property class="ModuleAdmin.lvclass"(reference=w205, error in=w199) -> (error out=w198:errorcluster, "Accessors:Module ID"=w204:i32)  [unwired: 1 out]
            n236 = call "StatusUpdate.vi"("error in (no error)"=w198, "Status"="Data Stopped", "ModuleID"=w204) -> ("error out"=w203:errorcluster)  [unwired: 8 in]
            n237 = call "SetGetState.vi"("Set (f)"=TRUE, "State In"=w201) -> ()  [unwired: 9 in, 1 out]
            n238 = call "Enqueue.vi"("MessageQueue"=w200, "Message"=w201, "error in (no error)"=w203, "Type of Enqueue"=enum16{"Else", "LE"}."LE" ("Enum")) -> ("error out"=w202:errorcluster)  [unwired: 10 in, 1 out]
          }
          frame "Exit" {
          }
        }
        n239 = call "ErrorHandler.vi"("error in (no error)"=w91, "MessageQueue"=w93) -> ("error out"=w92:errorcluster)  [unwired: 8 in, 1 out]
      }
    }
    frame Error {
      w727 = T6 2 items=["no dialog", "OK message", "continue or stop message", "OK message + warnings", "continue/stop + warnings"] ("type of dialog (OK msg:1)")
      n240 = property class="ModuleAdmin.lvclass"(reference=w734) -> (reference out=w732:refnum<class "ModuleAdmin.lvclass">, error out=w728:errorcluster, "Accessors:CloneRegRef"=w731:refnum<data-value>, "Accessors:Module ID"=w730:i32)  [unwired: 1 in]
      n241 = call <userlib>:"Remove.vi"("error in (no error)"=w728, "Module ID"=w730, "CloneRegRef"=w731) -> ("error out"=w736:errorcluster)  [unwired: 6 in, 2 out]
      n242 = flat-sequence {
        tunnel: w737 -> [w740]
        tunnel: w736 -> [_]
        tunnel: [w739] -> w735
        tunnel: w727 -> [w738]
        frame #0 {
          n243 = call <vilib>:"Simple Error Handler.vi"("type of dialog (OK msg:1)"=w738, "error in (no error)"=w740) -> ("error out"=w739:errorcluster)  [unwired: 3 in, 4 out]
        }
      }
    }
  }
  n244 = call "DestroyClone.vi"("error in (no error)"=w53, "Exit via Stop Module Req?"=w49, "Wait for Module to stop?"=w50, "ModuleAdmin"=w51) -> ("error out"=w52:errorcluster, "External Launch"=w48:bool)  [unwired: 5 in, 1 out]
  n245 = Unregister For Events(event registration refnum=w46, error in=w47) -> (error out=w45:errorcluster)
  n246 = Release Queue(queue=w58, force destroy? (F)=w16, error in (no error)=w52) -> (error out=w5:errorcluster)  [unwired: 2 out]
  n247 = Release Queue(queue=w18, force destroy? (F)=w16) -> (error out=w6:errorcluster)  [unwired: 1 in, 2 out]
  n248 = Release Queue(queue=w17, force destroy? (F)=w16) -> (error out=w7:errorcluster)  [unwired: 1 in, 2 out]
  n249 = Release Queue(queue=w10) -> (error out=w8:errorcluster)  [unwired: 2 in, 2 out]
  n250 = Merge Errors(w8, w7, w6, w5) -> (w9:errorcluster)
  n251 = Merge Errors(w45, w9, w27) -> (w37:errorcluster)
  n252 = case shown="True" w48 {
    tunnel: w37 -> [w741 w744]
    tunnel: [w741 w742] -> w36
    frame False {
    }
    frame True {
      n253 = control-ref of="This VI"() -> (w743:refnum<vi>)
      n254 = case shown="No Error" w744 {
        selector: w744 -> [w746 _]
        tunnel: w743 -> [w747 w749]
        tunnel: [w745 w748] -> w742
        frame No Error {
          n255 = invoke class="VI" method="FP.Close"(reference=w747, error in=w746) -> (error out=w745:errorcluster)  [unwired: 1 in, 2 out]
        }
        frame Error {
          n256 = invoke class="VI" method="FP.Open"(reference=w749, "Activate"=TRUE ("Activate?")) -> (error out=w748:errorcluster)  [unwired: 3 in, 4 out]
        }
      }
    }
  }
  "error out" <- w36
